vi "Tree Interaction.vi"() -> ()   [LabVIEW 2017, in "Tree API.lvlib" / "Tree.lvclass"]
uses:
  Tree.lvclass
  API/Set Attribute.vi
  API/Get Name.vi
  API/Get Attribute.vi
panel:
  out "Tag":string
  out "Attribute Value":variant
  out "Clicked Attribute Name":string
  out "Clicked Tree Name":string
  in  "Stop Button":bool
  in  "Tree":string(tree)
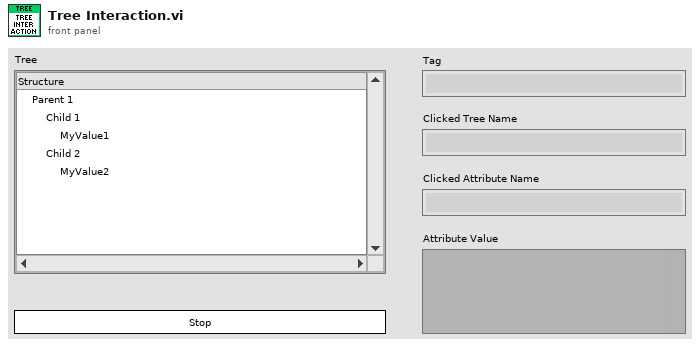
[diagram p1: front panel]
types:
  T1 = cluster{"Left Cell String":string, "Child Text":string[], "Child Tag":string, "Item Indent":i32, "Child Only?":bool, "Glyph Index":i32}[]
  T2 = typedef "LVPoint32TypeDef.ctl" = cluster{"Horizontal":i32, "Vertical":i32}
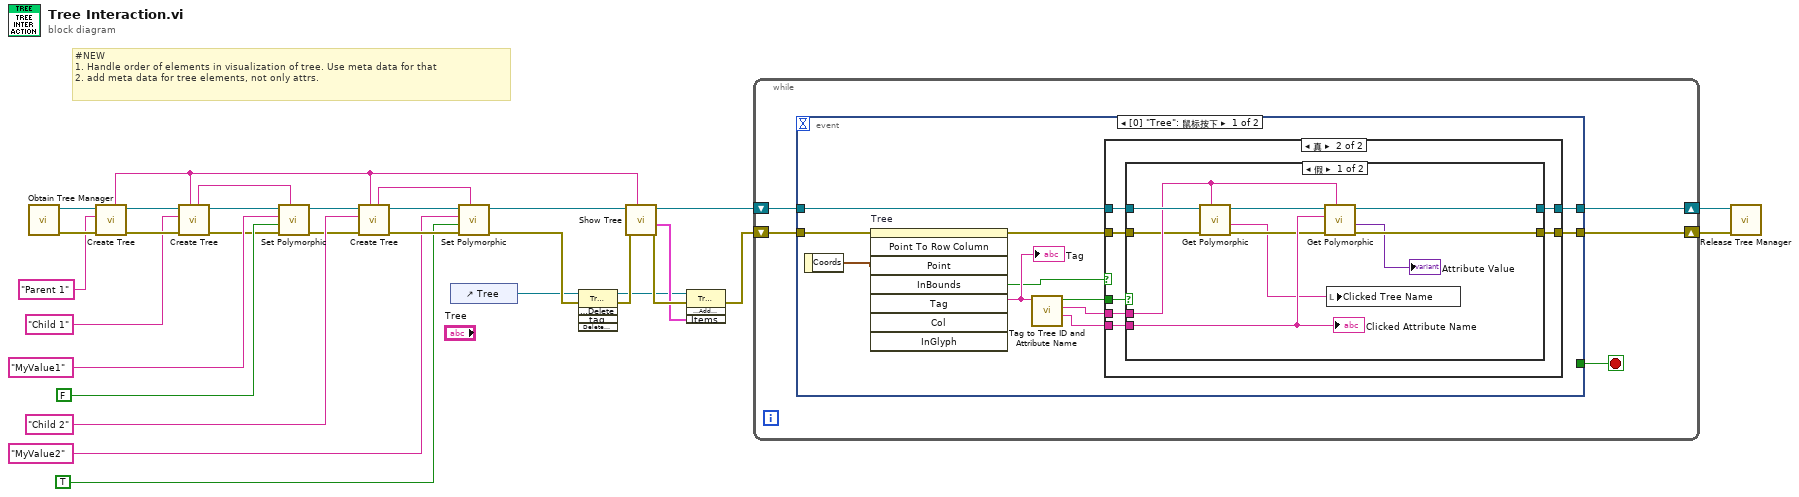
[diagram p0: block diagram]
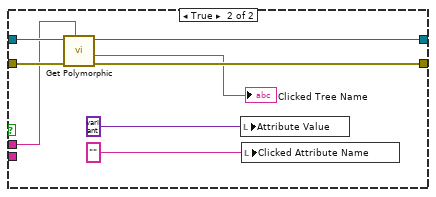
[diagram p3: hidden frame]
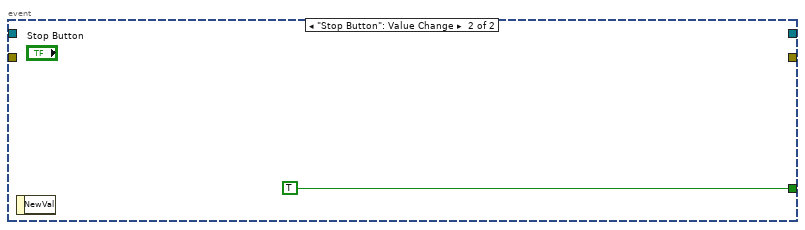
[diagram p4: hidden frame]
diagram:
  # "#NEW\n1. Handle order of elements in visualization of tree. Use meta data for that\n2. add meta data for tree elements, not only attrs."
  n1 = call "Obtain Tree Manager.vi"() -> ("Error Out"=w30:errorcluster, "Tree"=w31:refnum<data-value>)  [unwired: 10 in]
  n2 = call "Create Tree.vi"("Error In"=w30, "Name"="Parent 1", "Tree Manager"=w31) -> ("Error Out"=w28:errorcluster, "Tree Manager"=w29:refnum<data-value>, "Unique ID"=w10:string)  [unwired: 6 in]
  n3 = call "Create Tree.vi"("Parent ID (empty)"=w10, "Error In"=w28, "Name"="Child 1", "Tree Manager"=w29) -> ("Error Out"=w13:errorcluster, "Tree Manager"=w18:refnum<data-value>, "Unique ID"=w9:string)  [unwired: 5 in]
  n4 = call-poly "Set Polymorphic.vi"("Tree ID"=w9, "Error In"=w13, "Attribute Value"=FALSE, "Attribute Name"="MyValue1" ("Name"), "Tree Manager"=w18) -> ("Error Out"=w16:errorcluster, "Tree Manager"=w17:refnum<data-value>)  [unwired: 4 in, 1 out]
  n5 = call "Create Tree.vi"("Parent ID (empty)"=w10, "Error In"=w16, "Name"="Child 2", "Tree Manager"=w17) -> ("Error Out"=w22:errorcluster, "Tree Manager"=w23:refnum<data-value>, "Unique ID"=w8:string)  [unwired: 5 in]
  n6 = control-ref of="Tree"() -> (w2:refnum<vi>)
  n7 = call-poly "Set Polymorphic.vi"("Tree ID"=w8, "Error In"=w22, "Attribute Value"=TRUE, "Attribute Name"="MyValue2" ("Name"), "Tree Manager"=w23) -> ("Error Out"=w7:errorcluster, "Tree Manager"=w19:refnum<data-value>)  [unwired: 4 in, 1 out]
  n8 = invoke class="Tree (strict)" method="Edit Tree Items.Delete"(reference=w2, error in=w7) -> (reference out=w1:refnum<vi>, error out=w6:errorcluster)  [unwired: 3 in, 3 out]
  n9 = call "Show Tree.vi"("Root ID"=w10, "Error In"=w6, "Tree"=w19) -> ("Error Out"=w5:errorcluster, "Items Out"=w3:T1, "Tree"=w24:refnum<data-value>)  [unwired: 6 in]
  n10 = invoke class="Tree (strict)" method="Edit Tree Items.Add Multiple Items to End"(reference=w1, error in=w5, "Items"=w3) -> (error out=w4:errorcluster)  [unwired: 1 in, 3 out]
  n11 = while {
    shift-right: [w32] -> w12
    shift-left: w24 -> [w34]
    shift-right: [w33] -> w11
    shift-left: w4 -> [w35]
    stop <- w36 stop-if-true
    n12 = event shown="[0] \"Tree\": 鼠标按下" {
      selector: _ -> [_ _]
      dyn-events: _ -> [_ _]
      timeout: _ -> [_ _]
      tunnel: [_ TRUE] -> w36
      tunnel: w35 -> [w45 _]
      tunnel: w34 -> [w41 _]
      tunnel: [w39 _] -> w33
      tunnel: [w38 _] -> w32
      event "Tree": Mouse Down {
        n13 = event-data() -> ("Coords"=w47:T2)  [unwired: 1 in]
        n14 = invoke on="Tree" class="Tree (strict)" method="Point To Row Column"(error in=w45, "Point"=w47) -> (error out=w40:errorcluster, "InBounds"=w44:bool, "Tag"=w46:string)  [unwired: 6 in, 5 out]
        "Tag" <- w46
        n15 = call "Tag to Tree ID and Attribute Name.vi"("Tag"=w46) -> ("Attribute Name"=w37:string, "Tree ID"=w42:string, "Tree"=w43:bool)  [unwired: 8 in]
        n16 = case shown="真" w44 {
          tunnel: w43 -> [_ w56]
          tunnel: w42 -> [_ w55]
          tunnel: w41 -> [w49 w54]
          tunnel: w40 -> [w48 w53]
          tunnel: [w48 w52] -> w39
          tunnel: [w49 w51] -> w38
          tunnel: w37 -> [_ w50]
          frame False {
          }
          frame True {
            n17 = case shown="假" w56 {
              tunnel: w55 -> [w61 w69]
              tunnel: w54 -> [w62 w74]
              tunnel: w53 -> [w58 w73]
              tunnel: [w65 w72] -> w52
              tunnel: [w66 w71] -> w51
              tunnel: w50 -> [w63 _]
              frame False {
                n18 = call-poly "Get Polymorphic.vi"("Tree ID"=w61, "Error In"=w58, "Tree Manager"=w62) -> ("Error Out"=w59:errorcluster, "Name"=w57:string, "Tree Manager"=w60:refnum<data-value>)  [unwired: 6 in]
                n19 = call-poly "Get Polymorphic.vi"("Tree ID"=w61, "Error In"=w59, "Attribute Name"=w63, "Tree Manager"=w60) -> ("Error Out"=w65:errorcluster, "Attribute Value"=→"Attribute Value":variant, "Tree Manager"=w66:refnum<data-value>)  [unwired: 4 in, 1 out]
                n20 = local write "Clicked Tree Name"(w57) -> ()
                "Clicked Attribute Name" <- w63
              }
              frame True {
                n21 = call-poly "Get Polymorphic.vi"("Tree ID"=w69, "Error In"=w73, "Tree Manager"=w74) -> ("Error Out"=w72:errorcluster, "Name"=→"Clicked Tree Name":string, "Tree Manager"=w71:refnum<data-value>)  [unwired: 6 in]
                n22 = local write "Attribute Value"(variant) -> ()
                n23 = local write "Clicked Attribute Name"("" ("Clicked Attribute Name")) -> ()
              }
            }
          }
        }
      }
      event "Stop Button": Value Change {
        n24 = event-data() -> ()  [unwired: 1 in, 1 out]
      }
    }
  }
  n25 = call "Release Tree Manager.vi"("Error In"=w11, "Tree"=w12) -> ()  [unwired: 9 in, 1 out]
